vi "Adapt To Type.vi"(7 "Type and Defaults":variant, 8 "error in (no error)":errorcluster, 10 "Variant in":variant, 11 "Deserializer in":refnum<class "JSON Deserializer.lvclass">) -> (0 "error out":errorcluster, 2 "Variant out":variant, 3 "Deserializer out":refnum<class "JSON Deserializer.lvclass">)   [LabVIEW 2013, in "JKI JSON Serialization.lvlib" / "JSON Deserializer.lvclass"]
doc: "Adapts <b>Variant in</b> previously unflattened from a JSON formatted string to match the type of <b>Type and Defaults</b>. For any cluster element in Type and Defaults, the value of the element in Type and Default is used if element with the same name is not present in Variant in."
uses:
  JSON Deserializer.lvclass
  JSON Deserializer.lvclass/JSON Deserializer.ctl
  <vilib>/Utility/VariantDataType/VariantType.lvlib
  JKI JSON Serialization.lvlib
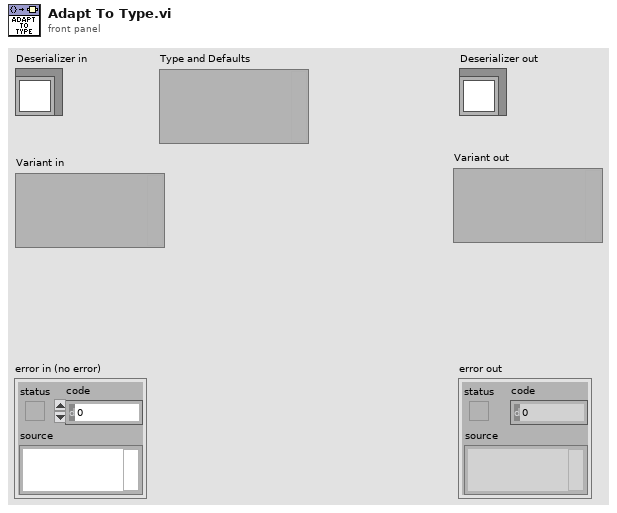
[diagram p1: front panel]
types:
  T1 = typedef "VariantType.lvlib/Type.ctl" = enum8{"Invalid Type", "Void", "I8", "I16", "I32", "I64", "U8", "U16", "U32", "U64", "Single Float", "Double Float", "Extended Float", "Single Complex", "Double Complex", "Extended Complex", "Enum U8", "Enum U16", "Enum U32", "Enum U64", "Single Float With Unit", "Double Float With Unit", "Extended Float With Unit", "Single Complex with Unit", "Double Complex with Unit", "Extended Complex with Unit", "Boolean", "String", "Path", "Picture", "Tag", "Array", "Cluster", "Variant", "LV Variant", "Waveform", "Timestamp", "Digital Waveform", "Digital Data", "ExpressData", "Refnum", "External Data", "VI", "Poly VI", "LabVIEW Class Instance", "Fixed Point"}
  T2 = typedef "VariantType.lvlib/MemoryInfo.ctl" = cluster{"Type":T3, "Size":u32}
  T3 = typedef "VariantType.lvlib/MemoryType.ctl" = enum16{"Variable", "Fixed", "Bounded"}
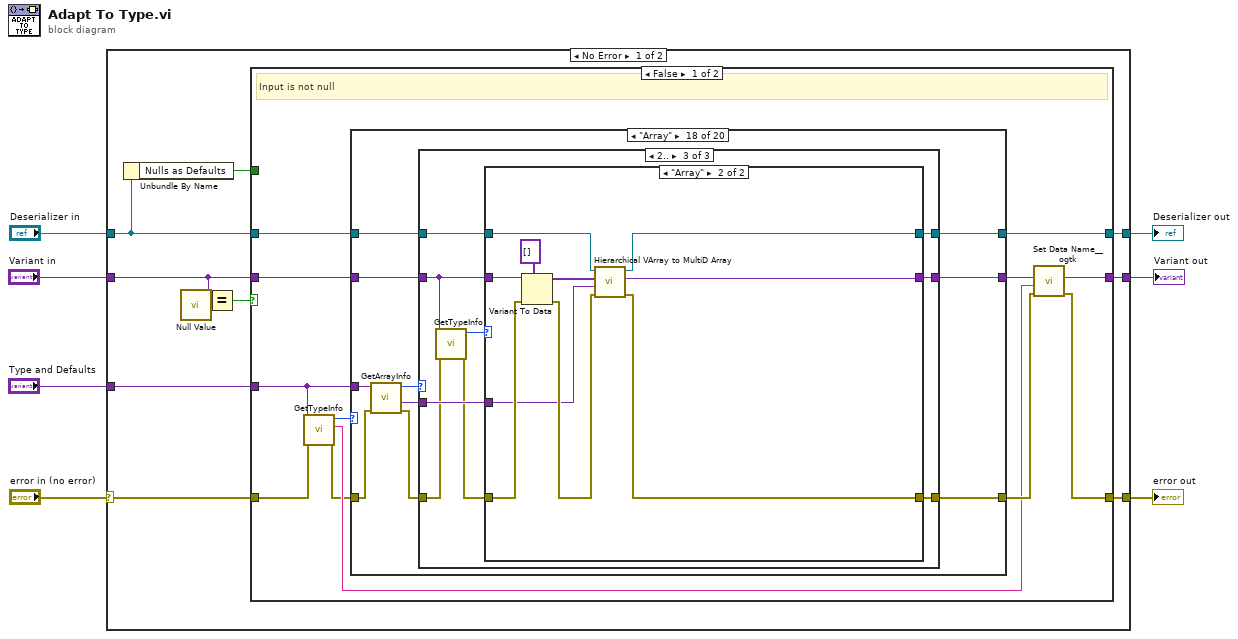
[diagram p0: block diagram]
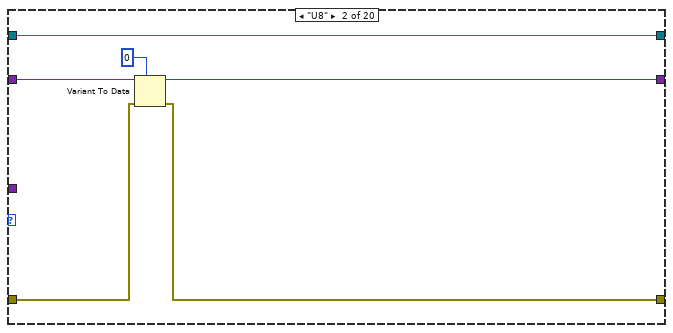
[diagram p3: hidden frame]
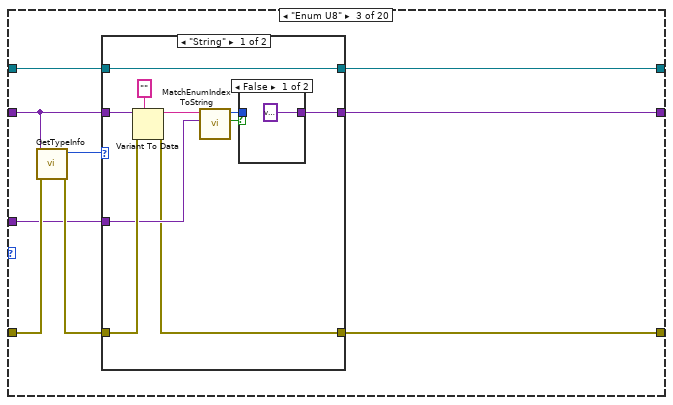
[diagram p4: hidden frame]
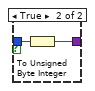
[diagram p5: hidden frame]
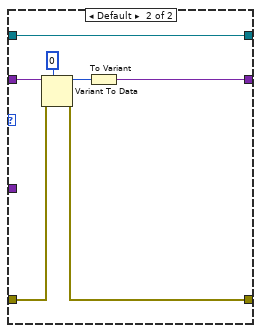
[diagram p6: hidden frame]
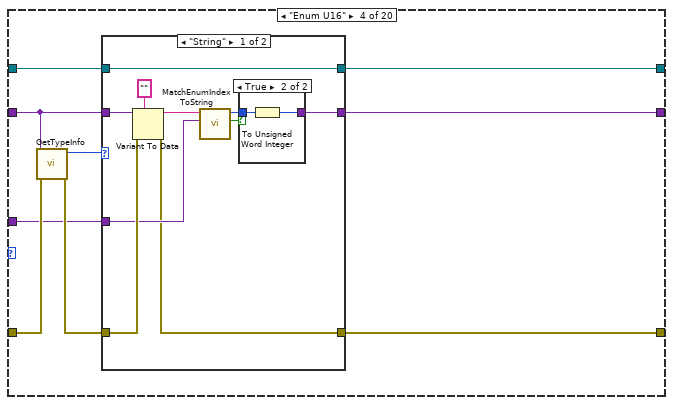
[diagram p7: hidden frame]
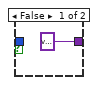
[diagram p8: hidden frame]
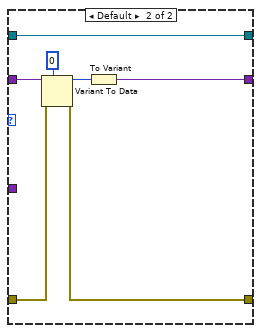
[diagram p9: hidden frame]
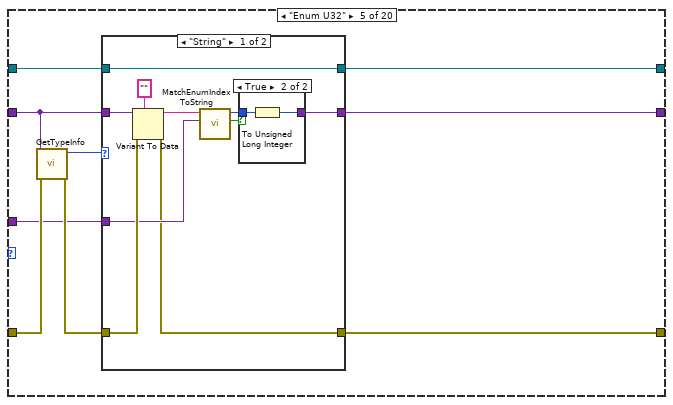
[diagram p10: hidden frame]
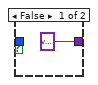
[diagram p11: hidden frame]
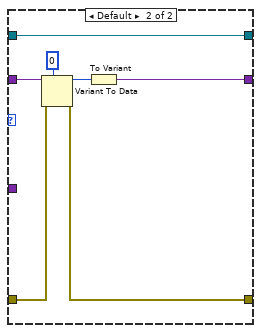
[diagram p12: hidden frame]
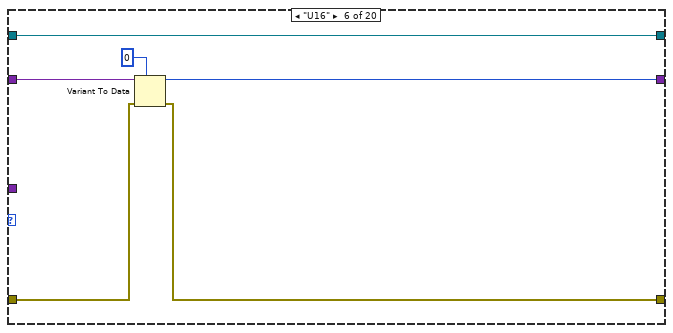
[diagram p13: hidden frame]
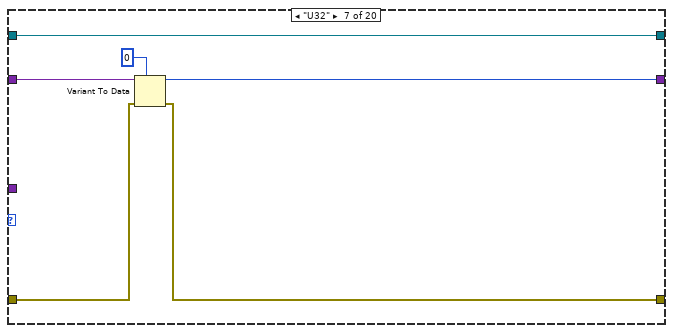
[diagram p14: hidden frame]
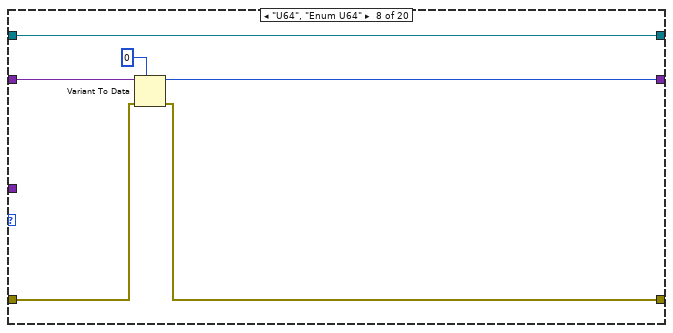
[diagram p15: hidden frame]
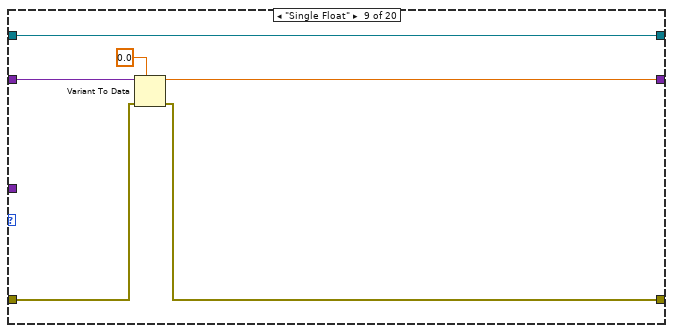
[diagram p16: hidden frame]
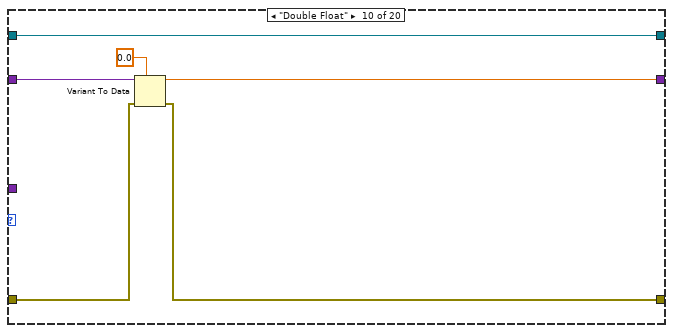
[diagram p17: hidden frame]
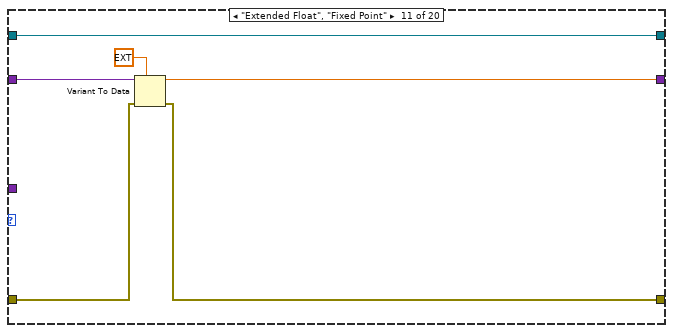
[diagram p18: hidden frame]
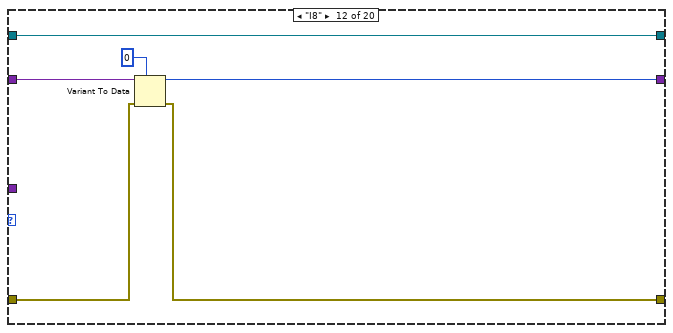
[diagram p19: hidden frame]
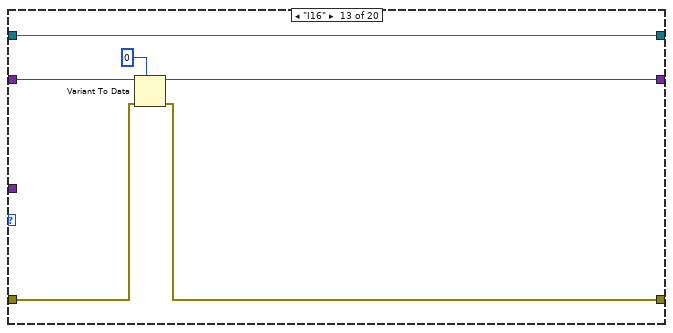
[diagram p20: hidden frame]
diagram:
  n1 = case shown="No Error" "error in (no error)" {
    selector: "error in (no error)" -> [w16 w435]
    tunnel: "Deserializer in" -> [w9 w436]
    tunnel: "Variant in" -> [w12 _]
    tunnel: [w13 w435] -> w4
    tunnel: "Type and Defaults" -> [w15 w434]
    tunnel: [w17 w436] -> w2
    tunnel: [w14 w434] -> w1
    frame No Error {
      n2 = Unbundle By Name(w9) -> ("Nulls as Defaults"=w8:bool)
      n3 = call "Null Value.vi"() -> ("Null"=w11:variant)
      n4 = Equal?(x=w12, y=w11) -> (x = y?=w10:bool)
      n5 = case shown="False" w10 {
        tunnel: w9 -> [w28 w375]
        tunnel: [w27 w374] -> w17
        tunnel: w16 -> [w26 w372]
        tunnel: w15 -> [w25 w376]
        tunnel: [w23 w377] -> w14
        tunnel: [w22 w371] -> w13
        tunnel: w12 -> [w18 w373]
        tunnel: w8 -> [_ w370]
        frame False {
          # "Input is not null"
          n6 = call <vilib>:"GetTypeInfo.vi"("error in (no error)"=w26, "Variant"=w25) -> ("error out"=w19:errorcluster, "Name"=w20:string, "Type Enum"=w29:T1)  [unwired: 5 in, 2 out]
          n7 = case shown="\"Array\"" w29 {
            tunnel: [w31 w35 w45 w74 w103 w128 w134 w140 w146 w152 w158 w164 w170 w176 w182 w191 w194 w207 w288 w367] -> w21
            tunnel: w19 -> [w31 w36 w43 w72 w101 w129 w135 w141 w147 w153 w159 w165 w171 w177 w183 w188 w198 w209 w287 w367]
            tunnel: w28 -> [w32 w38 w41 w70 w99 w131 w137 w143 w149 w155 w161 w167 w173 w179 w185 w192 w200 w206 w292 w369]
            tunnel: [w32 w38 w40 w69 w98 w131 w137 w143 w149 w155 w161 w167 w173 w179 w185 w192 w200 w204 w291 w369] -> w27
            tunnel: w25 -> [_ _ w39 w68 w97 _ _ _ _ _ _ _ _ _ _ _ _ w210 w290 _]
            tunnel: w18 -> [w30 w37 w46 w75 w104 w130 w136 w142 w148 w154 w160 w166 w172 w178 w184 w189 w199 w201 w285 w368]
            tunnel: [w30 w33 w47 w76 w105 w126 w132 w138 w144 w150 w156 w162 w168 w174 w180 w190 w193 w203 w289 w368] -> w24
            frame "Void", Default {
            }
            frame "U8" {
              n8 = Variant To Data(error in=w36, type=u8 0, Variant=w37) -> (data=w33:u8, error out=w35:errorcluster)
            }
            frame "Enum U8" {
              n9 = call <vilib>:"GetTypeInfo.vi"("error in (no error)"=w43, "Variant"=w46) -> ("error out"=w42:errorcluster, "Type Enum"=w44:T1)  [unwired: 5 in, 3 out]
              n10 = case shown="\"String\"" w44 {
                tunnel: [w51 w61] -> w47
                tunnel: w46 -> [w57 w65]
                tunnel: w42 -> [w55 w64]
                tunnel: [w48 w63] -> w45
                tunnel: w41 -> [w49 w62]
                tunnel: [w49 w62] -> w40
                tunnel: w39 -> [w53 _]
                frame "String" {
                  n11 = Variant To Data(error in=w55, type="", Variant=w57) -> (data=w54:string, error out=w48:errorcluster)
                  n12 = call "MatchEnumIndexToString.vi"("Enum Variant"=w53, "String"=w54) -> ("found"=w50:bool, "index"=w52:i32)  [unwired: 8 in]
                  n13 = case shown="False" w50 {
                    tunnel: w52 -> [_ w60]
                    tunnel: [variant ("Type and Defaults") w59] -> w51
                    frame False {
                    }
                    frame True {
                      n14 = To Unsigned Byte Integer(number=w60) -> (unsigned 8bit integer=w59:u8)
                    }
                  }
                }
                frame Default {
                  n15 = Variant To Data(error in=w64, type=u8 0, Variant=w65) -> (data=w66:u8, error out=w63:errorcluster)
                  n16 = To Variant(anything=w66) -> (Variant=w61:variant)
                }
              }
            }
            frame "Enum U16" {
              n17 = call <vilib>:"GetTypeInfo.vi"("error in (no error)"=w72, "Variant"=w75) -> ("error out"=w71:errorcluster, "Type Enum"=w73:T1)  [unwired: 5 in, 3 out]
              n18 = case shown="\"String\"" w73 {
                tunnel: [w80 w90] -> w76
                tunnel: w75 -> [w86 w94]
                tunnel: w71 -> [w84 w93]
                tunnel: [w77 w92] -> w74
                tunnel: w70 -> [w78 w91]
                tunnel: [w78 w91] -> w69
                tunnel: w68 -> [w82 _]
                frame "String" {
                  n19 = Variant To Data(error in=w84, type="", Variant=w86) -> (data=w83:string, error out=w77:errorcluster)
                  n20 = call "MatchEnumIndexToString.vi"("Enum Variant"=w82, "String"=w83) -> ("found"=w79:bool, "index"=w81:i32)  [unwired: 8 in]
                  n21 = case shown="True" w79 {
                    tunnel: w81 -> [_ w89]
                    tunnel: [variant ("Type and Defaults") w88] -> w80
                    frame False {
                    }
                    frame True {
                      n22 = To Unsigned Word Integer(number=w89) -> (unsigned 16bit integer=w88:u16)
                    }
                  }
                }
                frame Default {
                  n23 = Variant To Data(error in=w93, type=u16 0, Variant=w94) -> (data=w95:u16, error out=w92:errorcluster)
                  n24 = To Variant(anything=w95) -> (Variant=w90:variant)
                }
              }
            }
            frame "Enum U32" {
              n25 = call <vilib>:"GetTypeInfo.vi"("error in (no error)"=w101, "Variant"=w104) -> ("error out"=w100:errorcluster, "Type Enum"=w102:T1)  [unwired: 5 in, 3 out]
              n26 = case shown="\"String\"" w102 {
                tunnel: [w109 w119] -> w105
                tunnel: w104 -> [w115 w123]
                tunnel: w100 -> [w113 w122]
                tunnel: [w106 w121] -> w103
                tunnel: w99 -> [w107 w120]
                tunnel: [w107 w120] -> w98
                tunnel: w97 -> [w111 _]
                frame "String" {
                  n27 = Variant To Data(error in=w113, type="", Variant=w115) -> (data=w112:string, error out=w106:errorcluster)
                  n28 = call "MatchEnumIndexToString.vi"("Enum Variant"=w111, "String"=w112) -> ("found"=w108:bool, "index"=w110:i32)  [unwired: 8 in]
                  n29 = case shown="True" w108 {
                    tunnel: w110 -> [_ w118]
                    tunnel: [variant ("Type and Defaults") w117] -> w109
                    frame False {
                    }
                    frame True {
                      n30 = To Unsigned Long Integer(number=w118) -> (unsigned 32bit integer=w117:u32)
                    }
                  }
                }
                frame Default {
                  n31 = Variant To Data(error in=w122, type=u32 0, Variant=w123) -> (data=w124:u32, error out=w121:errorcluster)
                  n32 = To Variant(anything=w124) -> (Variant=w119:variant)
                }
              }
            }
            frame "U16" {
              n33 = Variant To Data(error in=w129, type=u16 0, Variant=w130) -> (data=w126:u16, error out=w128:errorcluster)
            }
            frame "U32" {
              n34 = Variant To Data(error in=w135, type=u32 0, Variant=w136) -> (data=w132:u32, error out=w134:errorcluster)
            }
            frame "U64", "Enum U64" {
              n35 = Variant To Data(error in=w141, type=u64 0, Variant=w142) -> (data=w138:u64, error out=w140:errorcluster)
            }
            frame "Single Float" {
              n36 = Variant To Data(error in=w147, type=sgl 0.0, Variant=w148) -> (data=w144:sgl, error out=w146:errorcluster)
            }
            frame "Double Float" {
              n37 = Variant To Data(error in=w153, type=0.0, Variant=w154) -> (data=w150:dbl, error out=w152:errorcluster)
            }
            frame "Extended Float", "Fixed Point" {
              n38 = Variant To Data(error in=w159, type=ext 0.0, Variant=w160) -> (data=w156:ext, error out=w158:errorcluster)
            }
            frame "I8" {
              n39 = Variant To Data(error in=w165, type=i8 0, Variant=w166) -> (data=w162:i8, error out=w164:errorcluster)
            }
            frame "I16" {
              n40 = Variant To Data(error in=w171, type=i16 0, Variant=w172) -> (data=w168:i16, error out=w170:errorcluster)
            }
            frame "I32" {
              n41 = Variant To Data(error in=w177, type=0, Variant=w178) -> (data=w174:i32, error out=w176:errorcluster)
            }
            frame "I64" {
              n42 = Variant To Data(error in=w183, type=i64 0, Variant=w184) -> (data=w180:i64, error out=w182:errorcluster)
            }
            frame "Path" {
              n43 = Variant To Data(error in=w188, type="", Variant=w189) -> (data=w186:string, error out=w191:errorcluster)
              n44 = String To Path(string=w186) -> (path=w190:path)
            }
            frame "Timestamp" {
              n45 = Variant To Data(error in=w198, type="", Variant=w199) -> (data=w196:string, error out=w195:errorcluster)
              n46 = call "ISO String To Timestamp.vi"("error in (no error)"=w195, "ISO Timestamp String"=w196) -> ("error out"=w194:errorcluster, "Time Stamp"=w193:timestamp)  [unwired: 8 in]
            }
            frame "Array" {
              n47 = call <vilib>:"GetArrayInfo.vi"("error in (no error)"=w209, "Variant"=w210) -> ("error out"=w208:errorcluster, "ArrayElement"=w205:variant, "NDims"=w202:i32)  [unwired: 6 in, 1 out]
              n48 = case shown="2.." w202 {
                tunnel: w208 -> [w213 w220 w265]
                tunnel: w201 -> [w215 w218 w263]
                tunnel: [w214 w225 w270] -> w207
                tunnel: w206 -> [w216 w224 w269]
                tunnel: w205 -> [_ w223 w268]
                tunnel: [w216 w222 w267] -> w204
                tunnel: [w215 w221 w266] -> w203
                frame 0, Default {
                  n49 = call <vilib>:"Error Cluster From Error Code.vi"("error in (no error)"=w213, "error message (\"\")"="Unflattening failed. Zero dimensional arrays not supported." ("error message (\"\")"), "error code (0)"=1) -> ("error out"=w214:errorcluster)  [unwired: 6 in]
                }
                frame 1 {
                  n50 = call <vilib>:"GetTypeInfo.vi"("error in (no error)"=w220, "Variant"=w218) -> ("error out"=w219:errorcluster, "Type Enum"=w217:T1)  [unwired: 5 in, 3 out]
                  n51 = case shown="\"Array\"" w217 {
                    tunnel: [w226 w236 w254] -> w225
                    tunnel: w224 -> [w228 w234 w253]
                    tunnel: w223 -> [w227 w233 w252]
                    tunnel: [w228 w232 w251] -> w222
                    tunnel: [w227 w231 w250] -> w221
                    tunnel: w219 -> [w226 w230 w247]
                    tunnel: w218 -> [_ w229 w249]
                    frame Default {
                    }
                    frame "Array" {
                      n52 = Variant To Data(error in=w230, type=variant[] [], Variant=w229) -> (data=w237:variant[], error out=w235:errorcluster)
                      n53 = for {
                        tunnel: w237 -> [w244] mode=indexing
                        shift-right: [w242] -> w236
                        shift-left: w235 -> [w243]
                        shift-right: [w240] -> w232
                        shift-left: w234 -> [w245]
                        tunnel: w233 -> [w241]
                        tunnel: [w239] -> w231 mode=indexing
                        n54 = call "Adapt To Type.vi"("Type and Defaults"=w241, "error in (no error)"=w243, "Variant in"=w244, "Deserializer in"=w245) -> ("error out"=w242:errorcluster, "Variant out"=w239:variant, "Deserializer out"=w240:refnum<class "JSON Deserializer.lvclass">)  [unwired: 5 in]
                      }
                    }
                    frame "Cluster" {
                      n55 = call <userlib>:"Cluster to Array of VData__ogtk.vi"("error in (no error)"=w247, "Cluster"=w249) -> ("error out"=w248:errorcluster, "Array of VData"=w246:variant[])  [unwired: 8 in]
                      n56 = for {
                        tunnel: w246 -> [w260] mode=indexing
                        shift-right: [w258] -> w254
                        shift-left: w248 -> [w259]
                        shift-right: [w256] -> w251
                        shift-left: w253 -> [w261]
                        tunnel: w252 -> [w257]
                        tunnel: [w255] -> w250 mode=indexing
                        n57 = call "Adapt To Type.vi"("Type and Defaults"=w257, "error in (no error)"=w259, "Variant in"=w260, "Deserializer in"=w261) -> ("error out"=w258:errorcluster, "Variant out"=w255:variant, "Deserializer out"=w256:refnum<class "JSON Deserializer.lvclass">)  [unwired: 5 in]
                      }
                    }
                  }
                }
                frame 2.. {
                  n58 = call <vilib>:"GetTypeInfo.vi"("error in (no error)"=w265, "Variant"=w263) -> ("error out"=w264:errorcluster, "Type Enum"=w262:T1)  [unwired: 5 in, 3 out]
                  n59 = case shown="\"Array\"" w262 {
                    tunnel: [w271 w278] -> w270
                    tunnel: w269 -> [w273 w275]
                    tunnel: w268 -> [w272 w276]
                    tunnel: [w273 w274] -> w267
                    tunnel: [w272 w277] -> w266
                    tunnel: w264 -> [w271 w282]
                    tunnel: w263 -> [_ w281]
                    frame Default {
                    }
                    frame "Array" {
                      n60 = Variant To Data(error in=w282, type=variant[] [], Variant=w281) -> (data=w280:variant[], error out=w279:errorcluster)
                      n61 = call "Hierarchical VArray to MultiD Array.vi"("error in (no error)"=w279, "Element Type"=w276, "Hierarchical Array"=w280, "Deserializer in"=w275) -> ("error out"=w278:errorcluster, "MultiD Array"=w277:variant, "Deserializer out"=w274:refnum<class "JSON Deserializer.lvclass">)  [unwired: 5 in]
                    }
                  }
                }
              }
            }
            frame "Cluster" {
              n62 = call <vilib>:"GetTypeInfo.vi"("error in (no error)"=w287, "Variant"=w285) -> ("error out"=w286:errorcluster, "Type Enum"=w284:T1)  [unwired: 5 in, 3 out]
              n63 = case shown="\"Void\"" w284 {
                tunnel: w292 -> [w298 w301 w307 w339]
                tunnel: [w298 w301 w306 w338] -> w291
                tunnel: w290 -> [w297 w300 w313 w337]
                tunnel: [w297 w300 w304 w329] -> w289
                tunnel: [w296 w299 w302 w326] -> w288
                tunnel: w286 -> [w295 w299 w312 w325]
                tunnel: w285 -> [_ _ w314 w324]
                frame "Invalid Type", Default {
                  n64 = call <vilib>:"Error Cluster From Error Code.vi"("error in (no error)"=w295, "error message (\"\")"="Cannot deserialize the input type into a cluster." ("error message (\"\")"), "error code (0)"=1) -> ("error out"=w296:errorcluster)  [unwired: 6 in]
                }
                frame "Void" {
                  # "Empty input object, use default values"
                }
                frame "Array" {
                  n65 = call <userlib>:"Cluster to Array of VData__ogtk.vi"("error in (no error)"=w312, "Cluster"=w313) -> ("error out"=w311:errorcluster, "Array of VData"=w310:variant[])  [unwired: 8 in]
                  n66 = call <userlib>:"Array to Array of VData__ogtk.vi"("error in (no error)"=w311, "MultiD Array"=w314) -> ("error out"=w308:errorcluster, "1D Array of Variants"=w309:variant[])  [unwired: 8 in]
                  n67 = for {
                    tunnel: w310 -> [w319] mode=indexing
                    tunnel: w309 -> [w322]
                    shift-right: [w317] -> w303
                    shift-left: w308 -> [w318]
                    shift-right: [w316] -> w306
                    shift-left: w307 -> [w323]
                    tunnel: [w315] -> w305 mode=indexing
                    i -> [w321]
                    n68 = Index Array(array=w322, index=w321) -> (element=w320:variant)
                    n69 = call "Adapt To Type.vi"("Type and Defaults"=w319, "error in (no error)"=w318, "Variant in"=w320, "Deserializer in"=w323) -> ("error out"=w317:errorcluster, "Variant out"=w315:variant, "Deserializer out"=w316:refnum<class "JSON Deserializer.lvclass">)  [unwired: 5 in]
                  }
                  n70 = call <userlib>:"Array of VData to VCluster__ogtk.vi"("error in (no error)"=w303, "Array"=w305) -> ("error out"=w302:errorcluster, "VCluster"=w304:variant)  [unwired: 8 in]
                }
                frame "Cluster" {
                  n71 = call <userlib>:"Cluster to Array of VData__ogtk.vi"("error in (no error)"=w325, "Cluster"=w337) -> ("error out"=w335:errorcluster, "Array of VData"=w336:variant[])  [unwired: 8 in]
                  n72 = call <userlib>:"Cluster to Array of VData__ogtk.vi"("error in (no error)"=w335, "Cluster"=w324) -> ("error out"=w331:errorcluster, "Array of VData"=w334:variant[])  [unwired: 8 in]
                  n73 = for {
                    tunnel: w334 -> [w341] mode=indexing
                    shift-right: [w342] -> w330
                    shift-left: w331 -> [w343]
                    tunnel: [w341] -> w333 mode=indexing
                    tunnel: [w340] -> w332 mode=indexing
                    n74 = call <vilib>:"GetTypeInfo.vi"("error in (no error)"=w343, "Variant"=w341) -> ("error out"=w342:errorcluster, "Name"=w340:string)  [unwired: 5 in, 3 out]
                  }
                  n75 = for {
                    shift-right: [w353] -> w327
                    shift-left: w330 -> [w348]
                    shift-right: [w352] -> w338
                    shift-left: w339 -> [w354]
                    tunnel: w336 -> [w345] mode=indexing
                    tunnel: [w351] -> w328 mode=indexing
                    tunnel: w333 -> [w346]
                    tunnel: w332 -> [w350]
                    n76 = call <vilib>:"GetTypeInfo.vi"("error in (no error)"=w348, "Variant"=w345) -> ("error out"=w347:errorcluster, "Name"=w349:string)  [unwired: 5 in, 3 out]
                    n77 = Search 1D Array(1D array=w350, element=w349) -> (index of element=w344:i32)  [unwired: 1 in]
                    n78 = case shown="0.." w344 {
                      selector: w344 -> [_ w358]
                      tunnel: w354 -> [w357 w366]
                      tunnel: [w355 w365] -> w353
                      tunnel: [w357 w364] -> w352
                      tunnel: [w356 w363] -> w351
                      tunnel: w347 -> [w355 w362]
                      tunnel: w346 -> [_ w361]
                      tunnel: w345 -> [w356 w359]
                      frame ..-1 {
                        # "Element not found"
                      }
                      frame 0.. {
                        # "Element found"
                        n79 = Index Array(array=w361, index=w358) -> (element=w360:variant)
                        n80 = call "Adapt To Type.vi"("Type and Defaults"=w359, "error in (no error)"=w362, "Variant in"=w360, "Deserializer in"=w366) -> ("error out"=w365:errorcluster, "Variant out"=w363:variant, "Deserializer out"=w364:refnum<class "JSON Deserializer.lvclass">)  [unwired: 5 in]
                      }
                    }
                  }
                  n81 = call <userlib>:"Array of VData to VCluster__ogtk.vi"("error in (no error)"=w327, "Array"=w328) -> ("error out"=w326:errorcluster, "VCluster"=w329:variant)  [unwired: 8 in]
                }
              }
            }
            frame "LV Variant" {
            }
          }
          n82 = call <userlib>:"Set Data Name__ogtk.vi"("error in (no error)"=w21, "Data Name"=w20, "Data"=w24) -> ("error out"=w22:errorcluster, "Renamed Data"=w23:variant)  [unwired: 7 in]
        }
        frame True {
          # "Input is null"
          n83 = case shown="False" w370 {
            tunnel: [w385 w433] -> w377
            tunnel: w376 -> [w382 w433]
            tunnel: w375 -> [w389 w432]
            tunnel: [w388 w432] -> w374
            tunnel: w373 -> [w387 _]
            tunnel: w372 -> [w381 w431]
            tunnel: [w383 w431] -> w371
            frame False {
              # "Return null value if supported by type"
              n84 = call <vilib>:"GetTypeInfo.vi"("error in (no error)"=w381, "Variant"=w382) -> ("error out"=w380:errorcluster, "Name"=w378:string, "Type Enum"=w379:T1)  [unwired: 5 in, 2 out]
              n85 = case shown="\"Array\"" w379 {
                tunnel: [w391 w393 w403] -> w384
                tunnel: w380 -> [w391 w393 w405]
                tunnel: w389 -> [w392 w395 w402]
                tunnel: [w392 w395 w400] -> w388
                tunnel: w382 -> [_ _ w406]
                tunnel: w387 -> [w390 _ w397]
                tunnel: [w390 path "" w399] -> w386
                frame Default {
                }
                frame "Path" {
                }
                frame "Array" {
                  n86 = call <vilib>:"GetArrayInfo.vi"("error in (no error)"=w405, "Variant"=w406) -> ("error out"=w404:errorcluster, "ArrayElement"=w401:variant, "Array Lengths"=w396:T2[], "NDims"=w398:i32)  [unwired: 6 in]
                  n87 = case shown="2.." w398 {
                    tunnel: w404 -> [w409 w416 w429]
                    tunnel: w397 -> [w411 _ _]
                    tunnel: [w410 w413 w423] -> w403
                    tunnel: w402 -> [w412 w417 w430]
                    tunnel: w401 -> [_ w415 w428]
                    tunnel: [w412 w417 w430] -> w400
                    tunnel: [w411 w418 w425] -> w399
                    tunnel: w396 -> [_ _ w422]
                    frame 0, Default {
                      n88 = call <vilib>:"Error Cluster From Error Code.vi"("error in (no error)"=w409, "error message (\"\")"="Unflattening failed. Zero dimensional arrays not supported." ("error message (\"\")"), "error code (0)"=1) -> ("error out"=w410:errorcluster)  [unwired: 6 in]
                    }
                    frame 1 {
                      n89 = call <userlib>:"Array of VData to VArray__ogtk.vi"("error in (no error)"=w416, "Element Type (when empty)"=w415, "1D Array of VData"=variant[] []) -> ("error out"=w413:errorcluster, "VArray"=w418:variant)  [unwired: 7 in]
                    }
                    frame 2.. {
                      n90 = Array Size(array=w422) -> (size(s)=w421:i32)
                      n91 = Initialize Array(0, w421) -> (w419:i32[])
                      n92 = call <userlib>:"Array of VData to VArray__ogtk.vi"("error in (no error)"=w429, "Element Type (when empty)"=w428, "1D Array of VData"=variant[] []) -> ("error out"=w424:errorcluster, "VArray"=w426:variant)  [unwired: 7 in]
                      n93 = call <userlib>:"Reshape 1D Array__ogtk.vi"("error in (no error)"=w424, "Size(s)"=w419, "1D Array"=w426) -> ("error out"=w423:errorcluster, "Reshaped VArray"=w425:variant)  [unwired: 7 in]
                    }
                  }
                }
              }
              n94 = call <userlib>:"Set Data Name__ogtk.vi"("error in (no error)"=w384, "Data Name"=w378, "Data"=w386) -> ("error out"=w383:errorcluster, "Renamed Data"=w385:variant)  [unwired: 7 in]
            }
            frame True {
              # "Return default value"
            }
          }
        }
      }
    }
    frame Error {
    }
  }
  "error out" <- w4
  "Deserializer out" <- w2
  "Variant out" <- w1
